vi "Nova_Postavka_Senzora.vi"() -> ()   [LabVIEW 2017]
uses:
  <vilib>/Waveform/WDTOps.llb/WDT Index Channel DBL.vi
panel:
  in  "Tab Control":enum32{"LIVE DATA", "Podesavanja"}(tab)
  out "Inteziteti ACC 1":waveform(dbl)(graph)
  out "Inteziteti ACC 2":waveform(dbl)(graph)
  out "Inteziteti ACC 3":waveform(dbl)(graph)
  out "TRENUTNI SIGNALI":dynamicdata(graph) caption="TRENUTNI SIGNALI !!!!"
  out "Iter":i32
  in  "File Name":string="LIVE_DATA"
  in  "Ponavljanja":i32=20
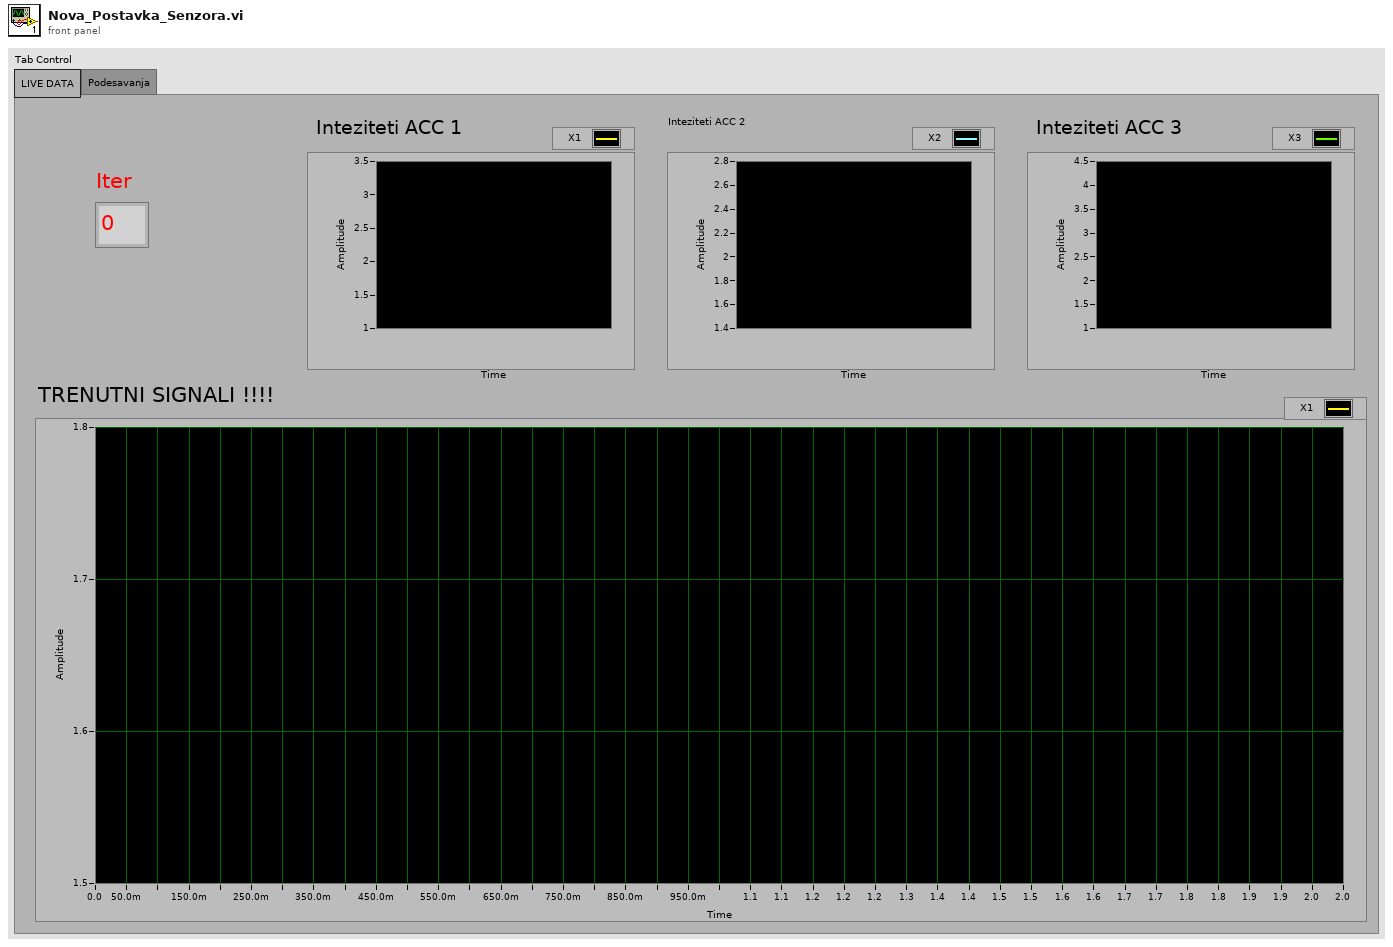
[diagram p1: front panel]
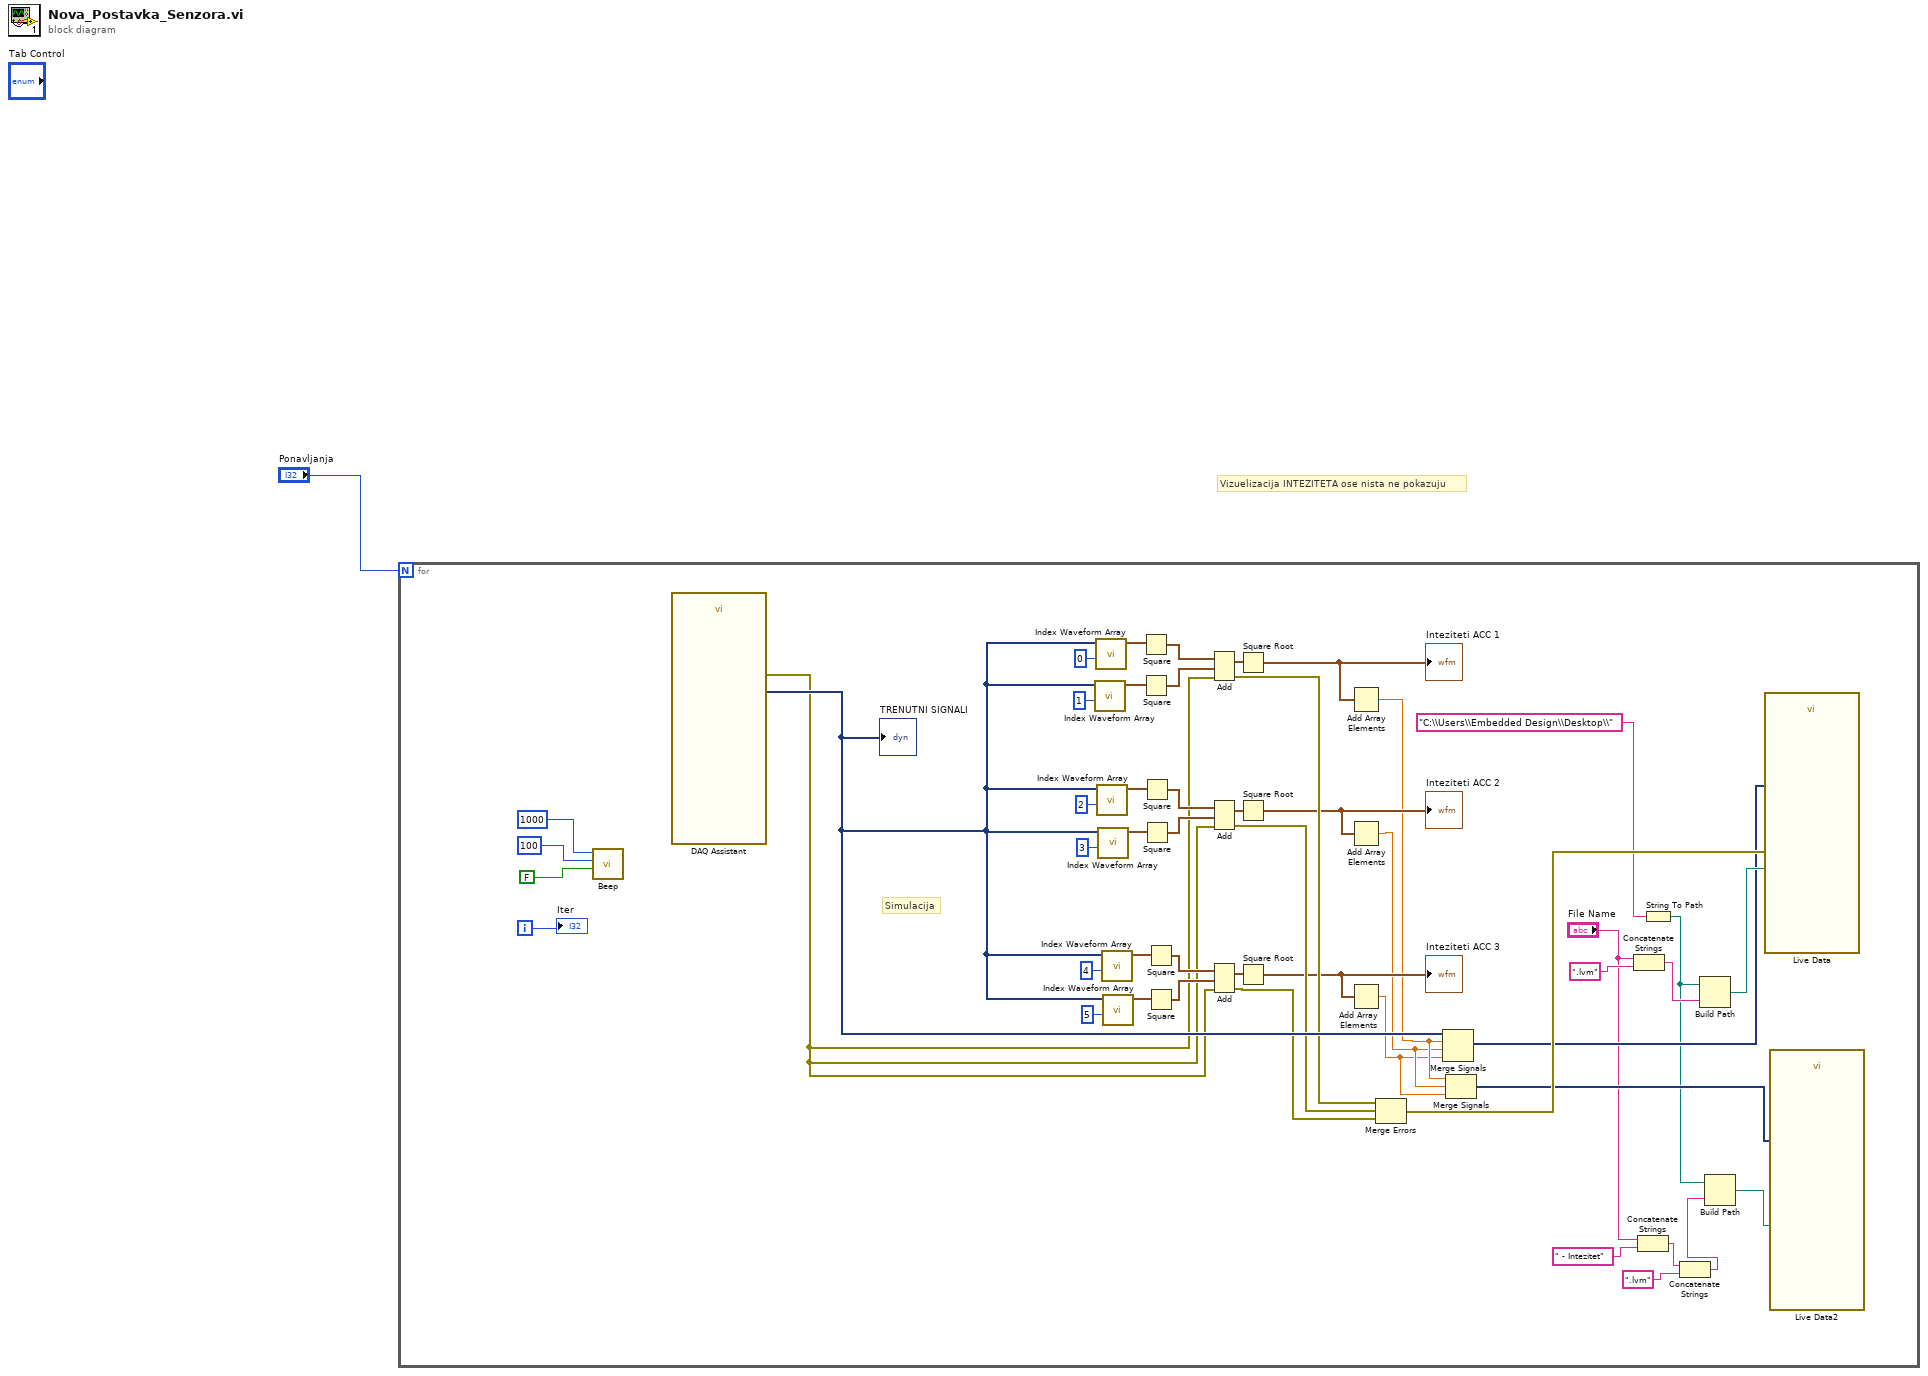
[diagram p0: block diagram]
diagram:
  # "Vizuelizacija INTEZITETA ose nista ne pokazuju"
  n1 = for {
    N: "Ponavljanja" -> [_]
    i -> [w13]
    # "Simulacija"
    n2 = call <vilib>:"Beep.vi"("use system alert? (T)"=FALSE, "duration (msec)"=u32 100, "frequency (Hz)"=u32 1000) -> ()  [unwired: 9 in]
    n3 = call "DAQ Assistant"() -> ("data"=w22:dynamicdata, "error out"=w21:errorcluster)  [unwired: 16 in, 2 out]
    "TRENUTNI SIGNALI" <- w22
    n4 = call-poly <vilib>:"Index Waveform Array.vi"("index"=1, "waveform array"=w22) -> ("waveform"=w36:waveform(dbl))  [unwired: 8 in, 1 out]
    n5 = call-poly <vilib>:"Index Waveform Array.vi"("index"=0, "waveform array"=w22) -> ("waveform"=w37:waveform(dbl))  [unwired: 8 in, 1 out]
    n6 = call-poly <vilib>:"Index Waveform Array.vi"("index"=2, "waveform array"=w22) -> ("waveform"=w35:waveform(dbl))  [unwired: 8 in, 1 out]
    n7 = call-poly <vilib>:"Index Waveform Array.vi"("index"=3, "waveform array"=w22) -> ("waveform"=w34:waveform(dbl))  [unwired: 8 in, 1 out]
    n8 = call-poly <vilib>:"Index Waveform Array.vi"("index"=4, "waveform array"=w22) -> ("waveform"=w33:waveform(dbl))  [unwired: 8 in, 1 out]
    n9 = call-poly <vilib>:"Index Waveform Array.vi"("index"=5, "waveform array"=w22) -> ("waveform"=w32:waveform(dbl))  [unwired: 8 in, 1 out]
    n10 = Square(x=w37) -> (x^2=w31:waveform(dbl))
    n11 = Square(x=w36) -> (x^2=w30:waveform(dbl))
    n12 = Square(x=w35) -> (x^2=w29:waveform(dbl))
    n13 = Square(x=w34) -> (x^2=w28:waveform(dbl))
    n14 = Square(x=w33) -> (x^2=w27:waveform(dbl))
    n15 = Square(x=w32) -> (x^2=w26:waveform(dbl))
    n16 = Add(1:w30, 2:w31, 4:w21) -> (0:w25:waveform(dbl), 3:w20:errorcluster)
    n17 = Add(1:w28, 2:w29, 4:w21) -> (0:w24:waveform(dbl), 3:w19:errorcluster)
    n18 = Add(1:w26, 2:w27, 4:w21) -> (0:w23:waveform(dbl), 3:w18:errorcluster)
    n19 = Square Root(x=w25) -> (sqrt(x)=w17:waveform(dbl))
    "Inteziteti ACC 1" <- w17
    n20 = Square Root(x=w24) -> (sqrt(x)=w16:waveform(dbl))
    "Inteziteti ACC 2" <- w16
    n21 = Square Root(x=w23) -> (sqrt(x)=w15:waveform(dbl))
    "Inteziteti ACC 3" <- w15
    n22 = Add Array Elements(numeric array=w17) -> (sum=w12:dbl)
    n23 = Add Array Elements(numeric array=w16) -> (sum=w11:dbl)
    n24 = Add Array Elements(numeric array=w15) -> (sum=w10:dbl)
    n25 = Merge Errors(w20, w19, w18) -> (w48:errorcluster)
    n26 = Merge Signals(w22, w12, w11, w10) -> (w14:dynamicdata)
    n27 = Merge Signals(w12, w11, w10) -> (w9:dynamicdata)
    n28 = Concatenate Strings("File Name", ".lvm" ("name or relative path")) -> (w44:string)
    n29 = Concatenate Strings("File Name", " - Intezitet" ("name or relative path")) -> (w6:string)
    n30 = String To Path(string="C:\\Users\\Embedded Design\\Desktop\\") -> (path=w4:path)
    n31 = Concatenate Strings(w6, ".lvm" ("name or relative path")) -> (w3:string)
    n32 = Build Path(base path=w4, name or relative path=w44) -> (appended path=w47:path)
    n33 = Build Path(base path=w4, name or relative path=w3) -> (appended path=w2:path)
    n34 = call "Live Data"("Signals"=w14, "error in (no error)"=w48, "Filename"=w47) -> ()  [unwired: 14 in, 3 out]
    n35 = call "Live Data2"("Signals"=w9, "Filename"=w2) -> ()  [unwired: 15 in, 3 out]
    "Iter" <- w13
  }
